vi "moment.vi"() -> ()   [LabVIEW 2022 SP3]
panel:
  in  "length 2":dbl[](array[numeric])=[44.0, 48.0, 64.0, 159.0, 244.0, 264.0, 271.0, 180.0] format="%.2f"
  in  "weight 2":dbl[](array[numeric])=[7.0, 0.75, 1.0, 1.25, 2.25, 3.0, 0.0, -5.0] format="%.2f"
  out "total weight":dbl format="%.2f"
  out "total moment":dbl format="%.2f"
  in  "length":dbl[](array[numeric])=[4.0, 20.0, 115.0, 200.0, 220.0, 315.0, 0.0, 0.0] format="%.2f"
  in  "weight":dbl[](array[numeric])=[0.75, 1.0, 1.25, 2.25, 3.0, -2.0, 0.0, 0.0] format="%.2f"
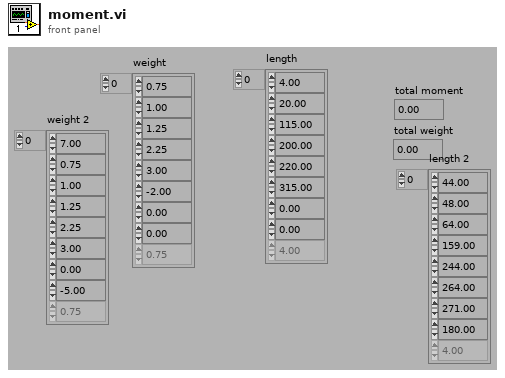
[diagram p1: front panel]
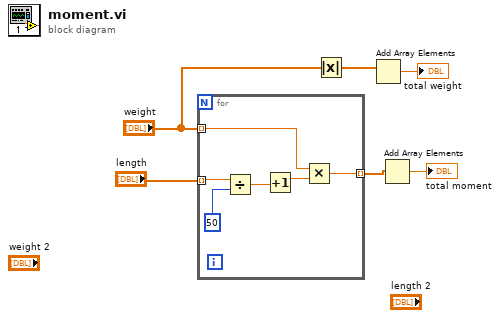
[diagram p0: block diagram]
diagram:
  n1 = for {
    tunnel: "length" -> [w12] mode=indexing
    tunnel: "weight" -> [w8] mode=indexing
    tunnel: [w7] -> w5 mode=indexing
    n2 = Divide(x=w12, y=50) -> (x/y=w10:dbl)
    n3 = Increment(x=w10) -> (x+1=w9:dbl)
    n4 = Multiply(x=w8, y=w9) -> (x*y=w7:dbl)
  }
  n5 = Absolute Value(x="weight") -> (abs(x)=w1:dbl[])
  n6 = Add Array Elements(numeric array=w1) -> (sum=→"total weight":dbl)
  n7 = Add Array Elements(numeric array=w5) -> (sum=→"total moment":dbl)
